vi "CO2FIX_GB19_Add455.vi"() -> ()   [LabVIEW 2018]
uses:
  <vilib>/DAQmx/read.llb/DAQmx Read (Analog DBL 1Chan 1Samp).vi
  <vilib>/DAQmx/create/channels.llb/DAQmx Create Channel (AI-Voltage-Basic).vi
  <vilib>/DAQmx/miscellaneous.llb/DAQmx Fill In Error Info.vi
  <vilib>/Utility/file.llb/Write Delimited Spreadsheet (DBL).vi
panel:
  out "Trans (Signal >275nm is more stable)":cluster{"Lumda":sgl[], "Intensity":sgl[]}(graph)
  out "< Thres":bool=TRUE
  out "number":u32=170738
  out "String":string="170738\r\n"
  out "Raw Data Graph 3":cluster{"Lumda":sgl[], "Intensity":sgl[]}(graph)
  in  "Save File":bool=TRUE
  in  "Save Background":bool
  out "> Thres":bool
  in  "stop":bool
  in  "Integration Time(ms)":i32=110
  in  "Average Times":i32=4
  in  "Wait Time":u32=120
  in  "UV300 Set":sgl=292000.0
  in  "UV340 Set":sgl=110378.0
  in  "Save ALL":bool=TRUE
  in  "file path (dialog if empty)":path=path "C:/Users/user/Desktop/CO2_Program/Data/0309/W_andMcd_New"
  in  "file path (dialog if empty) 2":path=path "C:/Users/user/Desktop/CO2_Program/Data/0309/W_and_Mcd_All_New"
  in  "Rate (ml/min)":dbl=0.003
  out "Dose Number":i32=1198
  in  "Pump Time":u32=1000
  out "Index":dbl=360.0
  in  "Wavelength":dbl=455.0
  in  "Pump RUN":bool
  in  "Connect the Pump":bool
  in  "Setting Tab":enum32{"UV and PL", "Range"}(tab)
  out "UV300":sgl(graph)=185217.0
  out "UV340":sgl(graph)=27758.75
  out "?":sgl=185217.0
  out "?":sgl=27758.75
  out "PL":dbl(graph)=0.15369048184948042
  out "?":dbl=0.15369048184948042 format="%0.2f"
  out "UV455 2":sgl=385808.3
  out "UV455":sgl(graph)=385808.3
  in  "Initial Wavelength 2":dbl=275.0
  out "Index 2":dbl=125.0
  in  "Final Wavelength":dbl=505.0
  out "Index 3":dbl=426.0
  out "subarray 2":sgl[](array[numeric])=[332.8669, 333.6288, 334.39072, 335.15262, 335.9145, 336.67633, 337.43814, 338.19995, 338.96173, 339.72348, 340.4852, 341.24692, 342.0086, 342.77026, 343.53192, 344.29355, 345.05515, 345.8167, 346.57825, 347.33978, 348.10126, 348.86273, 349.6242, 350.38562, 351.147, 351.9084]
  out "subarray":sgl[](array[numeric])=[290.1744, 290.93707, 291.6997, 292.46237, 293.225, 293.98764, 294.75027, 295.5129, 296.2755, 297.03812, 297.80072, 298.56332, 299.3259, 300.08847, 300.851, 301.6136, 302.37613, 303.13864, 303.90118, 304.6637, 305.42618, 306.1887, 306.95117, 307.71362, 308.47607, 309.23853]
  in  "index":i32=145
  in  "length 3":i32=26
  in  "index 2":i32=201
  in  "physical channels":tag="myDAQ1/ai0"
  out "Background":sgl[](graph)=[11662.829, 12200.412, 12741.526, 13266.624, 13764.132, 14239.703, 14700.305, 15169.1, 15633.125, 16080.848, 16526.568, 16951.803, 17352.846, 17742.307, 18115.617, 18481.635, 18861.121, 19228.037, 19607.826, 20033.656, 20506.39, 20975.314, 21429.824, 21874.693, 22314.486, 22720.926, 23099.477, 23464.29, 23812.91, 24120.67, 24402.24, 24671.984, 24942.217, 25128.393, 25328.764, 25352.076, 25260.271, 25075.955, 24881.014, 24785.152, 24827.955, 24950.078, 25146.15, 25347.043, 25523.666, 25693.074, 25799.213, 25776.885, 25635.168, 25390.854, 25115.197, 24923.48, 24850.783, 24866.639, 24948.094, 24974.553, 24984.9, 24962.344, 24914.252, 24755.438, 24523.752, 24313.99, 24132.727, 23955.791, 23793.834, 23694.123, 23663.645, 23690.838, 23774.723, 23913.729, 24066.088, 24197.506, 24283.953, 24334.453, 24349.229, 24376.02, 24419.385, 24459.86, 24472.574, 24419.55, 24302.516, 24156.85, 24001.873, 23888.658, 23819.984, 23787.754, 23826.557, 23969.12, 24233.43, 24581.705, 24935.51, 25101.64, 25095.82, 25118.697, 25217.166, 25398.553, 25656.426, 25987.393, 26384.482, 26612.795, 26693.918, 26686.576, 26673.998, 26773.516, 27020.361, 27379.266, 27767.031, 28061.688, 28225.52, 28304.275, 28338.377, 28412.365, 28553.605, 28743.72, 28936.129, 29089.033, 29184.336, 29222.68, 29278.357, 29416.11, 29634.06, 29921.674, 30173.553, 30232.85, 30100.656, 29836.76, 29570.885, 29519.438, 29756.2, 30166.668, 30678.26, 31253.81, 31798.094, 32115.113, 32270.998, 32535.479, 32940.16, 33297.176, 33591.727, 33730.51, 33711.863, 33752.2, 33593.383, 33535.496, 33506.03, 33496.426, 33561.37, 33725.746, 34031.348, 34486.812, 34979.957, 35071.03, 34906.305, 35122.027, 35674.387, 36218.492, 36514.16, 36119.66, 35296.406, 34884.29, 35104.91, 35851.824, 36744.855, 37013.312, 36519.266, 35533.914, 34533.707, 33783.926, 33529.125, 33507.043, 33761.26, 34125.36, 34354.758, 33803.387, 32718.762, 32014.986, 31773.3, 32030.799, 31726.107, 31596.922, 31384.887, 31393.861, 31548.842, 31469.758, 31146.816, 30741.807, 30337.123, 30063.309, 29974.361, 29922.512, 30067.191, 30719.6, 31695.77, 32920.945, 33695.24, 33394.07, 32401.562, 31569.3, 30980.309, 30304.057, 29715.104, 29526.53, 29929.428, 31339.666, 33072.6, 33885.43, 33322.734, 31445.363, 30226.885, 30152.033, 30646.63, 30937.982, 30534.053, 30046.96, 29539.832, 29029.887, 28704.307, 28765.17, 29236.066, 30154.299, 31222.639, 31898.865, 32050.398, 31853.746, 31434.635, 30982.043, 30593.57, 30154.084, 29726.898, 29487.102, 29371.229, 29195.447, 28703.057, 28216.209, 27783.318, 27229.06, 26700.953, 26456.951, 26509.146, 26732.828, 26917.287, 27316.756, 27877.488, 28221.094, 28203.2, 27723.234, 26970.273, 25911.797, 25373.816, 25795.814, 26985.47, 27935.127, 28164.598, 27135.84, 25322.652, 23791.945, 22817.662, 21753.3, 20725.24, 20196.85, 20215.668, 20613.348, 21187.29, 21629.316, 21783.09, 21561.031, 21078.72, 20720.355, 20649.633, 20746.46, 20994.38, 21363.48, 21437.719, 21286.775, 21083.664, 20873.533, 22341.213, 30386.02, 42265.0, 47372.523, 43005.14, 30858.705, 22305.854, 19230.033, 18336.748, 18041.25, 17642.873, 17564.633, 17787.107, 17785.61, 17619.354, 17703.818, 17906.27, 17665.78, 17110.701, 16657.889, 16782.773, 16929.34, 17048.264, 17154.547, 17162.465, 17056.4]
  in  "index 3":i32=355
  in  "length":i32=15
  out "subarray 3":sgl[](array[numeric])=[449.83356, 450.5899, 451.34622, 452.1025, 452.8587, 453.6149, 454.371, 455.12708, 455.8831, 456.63907, 457.395, 458.15088, 458.9067, 459.66248, 460.4182]
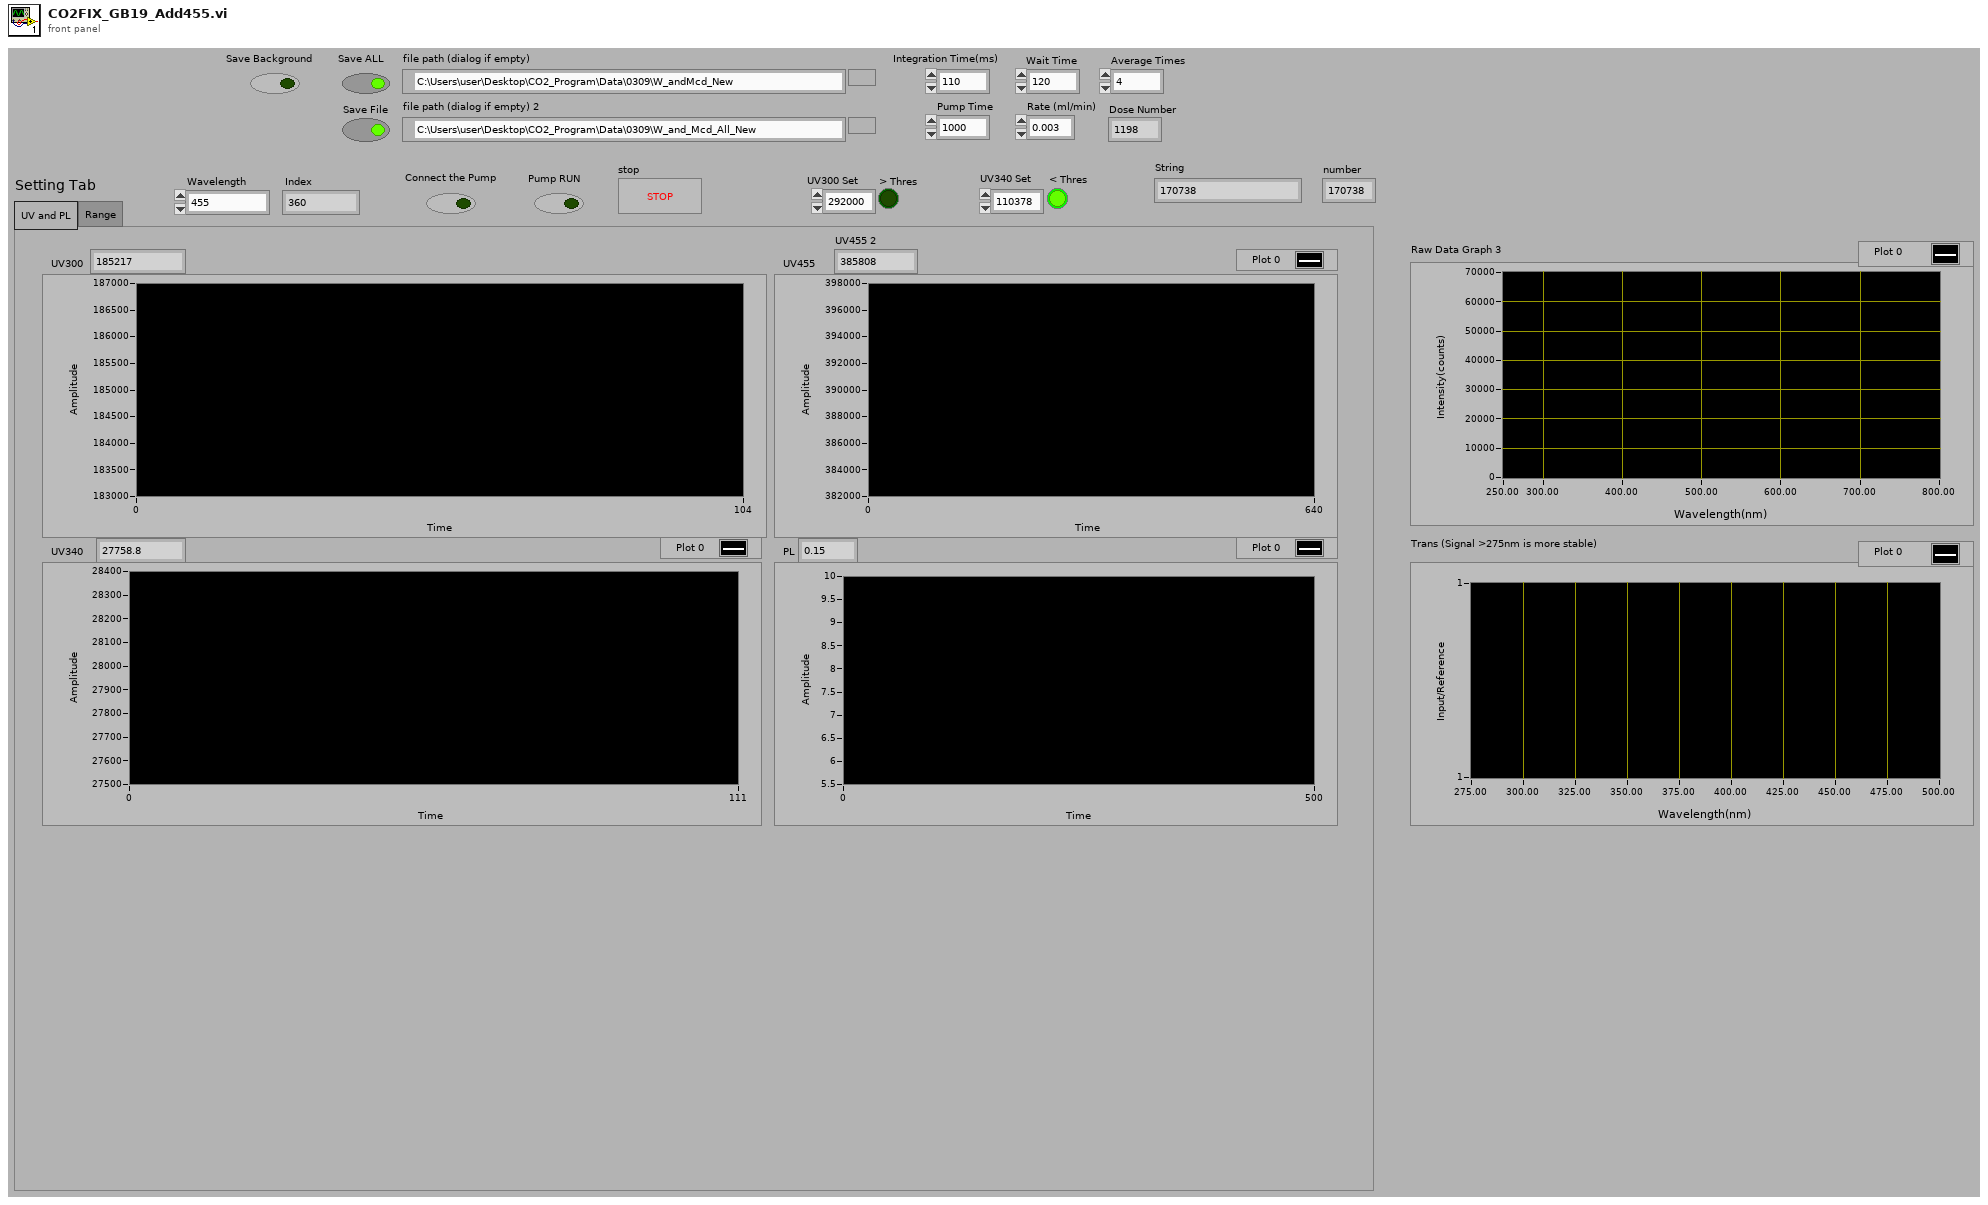
[diagram p1: front panel]
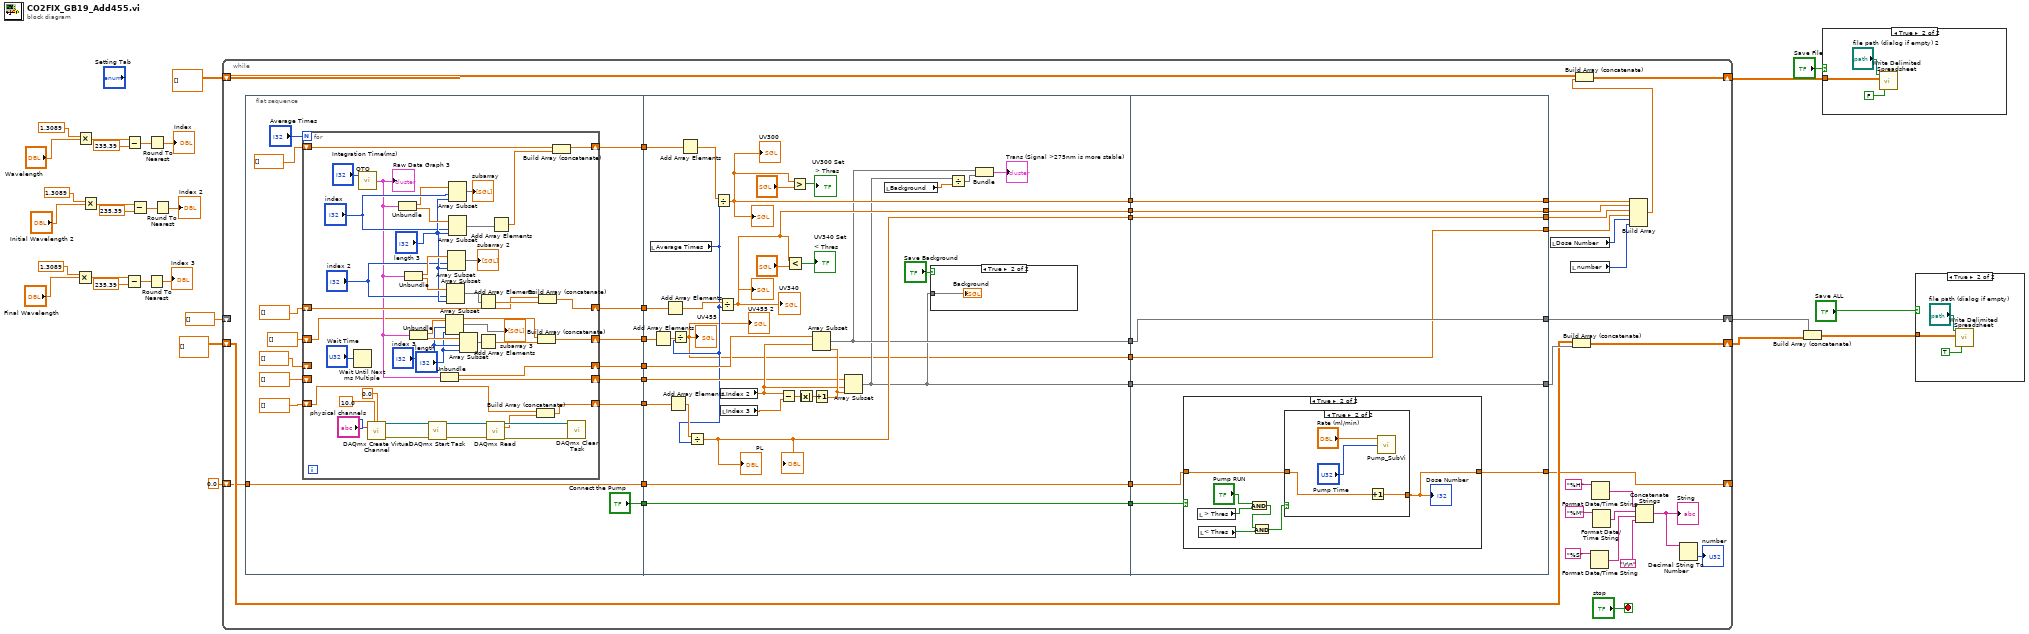
[diagram p0: block diagram]
diagram:
  n1 = Multiply(x=1.3089, y="Final Wavelength") -> (x*y=w12:dbl)
  n2 = Multiply(x=1.3089, y="Wavelength") -> (x*y=w27:dbl)
  n3 = Multiply(x=1.3089, y="Initial Wavelength 2") -> (x*y=w18:dbl)
  n4 = Subtract(x=w12, y=235.39) -> (x-y=w11:dbl)
  n5 = Subtract(x=w27, y=235.39) -> (x-y=w26:dbl)
  n6 = Subtract(x=w18, y=235.39) -> (x-y=w17:dbl)
  n7 = Round To Nearest(number=w11) -> (nearest integer value=→"Index 3":dbl)
  n8 = Round To Nearest(number=w26) -> (nearest integer value=→"Index":dbl)
  n9 = Round To Nearest(number=w17) -> (nearest integer value=→"Index 2":dbl)
  n10 = while {
    shift-right: [w49] -> w3
    shift-left: sgl[][] [] -> [w47]
    shift-right: [w55] -> w20
    shift-left: sgl[][] [] -> [w69]
    shift-right: [w48] -> w4
    shift-left: sgl[] [] -> [_]
    shift-right: [w46] -> _
    shift-left: 0.0 -> [w45]
    stop <- "stop" stop-if-true
    n11 = flat-sequence {
      tunnel: [w78] -> w67
      tunnel: [w77] -> w66
      tunnel: [w76] -> w65
      tunnel: ["Connect the Pump"] -> w61
      tunnel: [w74] -> w54
      tunnel: [w73] -> w53
      tunnel: w45 -> [w72]
      tunnel: [w72] -> w44
      tunnel: [w70] -> w33
      tunnel: w67 -> [w146]
      tunnel: w66 -> [w145]
      tunnel: w65 -> [w144]
      tunnel: [w148] -> w64
      tunnel: [w147] -> w63
      tunnel: [w143] -> w62
      tunnel: w61 -> [w143]
      tunnel: [w142] -> w58
      tunnel: w54 -> [w141]
      tunnel: w53 -> [w140]
      tunnel: [w134] -> w51
      tunnel: [w136] -> w50
      tunnel: w44 -> [w139]
      tunnel: [w139] -> w43
      tunnel: w33 -> [w131]
      tunnel: [w128] -> w30
      tunnel: [w168] -> w60
      tunnel: [w169] -> w59
      tunnel: w64 -> [w169]
      tunnel: w63 -> [w168]
      tunnel: w62 -> [w167]
      tunnel: [w166] -> w57
      tunnel: w58 -> [w166]
      tunnel: [w165] -> w52
      tunnel: w51 -> [w165]
      tunnel: w50 -> [w164]
      tunnel: [w164] -> w48
      tunnel: [w163] -> w46
      tunnel: w43 -> [w162]
      tunnel: w30 -> [w161]
      tunnel: [w161] -> w29
      frame #0 {
        n12 = for {
          N: "Average Times" -> [_]
          shift-right: [w121] -> w78
          shift-left: sgl[] [] -> [w120]
          shift-right: [w117] -> w76
          shift-left: sgl[] [] -> [w116]
          shift-right: [w113] -> w73
          shift-left: sgl[] [] ("Intensity") -> [_]
          shift-right: [w112] -> w74
          shift-left: sgl[] [] -> [_]
          shift-right: [w96] -> w77
          shift-left: dbl[] [] -> [w95]
          shift-right: [w90] -> w70
          shift-left: sgl[] [] -> [w89]
          n13 = Wait Until Next ms Multiple(millisecond multiple="Wait Time") -> ()  [unwired: 1 out]
          n14 = call "OTO.vi"("Integration Time(ms)"="Integration Time(ms)") -> ("Raw Data Graph"=w93:cluster{"Lumda":sgl[], "Intensity":sgl[]})  [unwired: 2 in]
          "Raw Data Graph 3" <- w93
          n15 = call-poly <vilib>:"DAQmx Create Virtual Channel.vi"("maximum value"=10.0, "minimum value"=0.0, "physical channels"="physical channels") -> ("task out"=w104:refnum<k21>, "error out"=w101:errorcluster)  [unwired: 11 in]
          n16 = Unbundle(w93) -> ("Lumda"=w109:sgl[], "Intensity"=w126:sgl[])
          n17 = Unbundle(w93) -> ("Lumda"=w125:sgl[], "Intensity"=w124:sgl[])
          n18 = Unbundle(w93) -> ("Lumda"=w87:sgl[], "Intensity"=w92:sgl[])
          n19 = call <vilib>:"DAQmx Start Task.vi"("task/channels in"=w104, "error in"=w101) -> ("task out"=w105:refnum<k21>, "error out"=w102:errorcluster)  [unwired: 12 in]
          n20 = Unbundle(w93) -> ("Lumda"=w112:sgl[], "Intensity"=w113:sgl[])
          n21 = Array Subset(array=w87, index="index 3", length="length") -> (→"subarray 3":sgl[])
          n22 = Array Subset(array=w124, index="index 2", length="length 3") -> (w114:sgl[])
          n23 = Array Subset(array=w125, index="index 2", length="length 3") -> (→"subarray 2":sgl[])
          n24 = Array Subset(array=w126, index="index", length="length 3") -> (w119:sgl[])
          n25 = Array Subset(array=w109, index="index", length="length 3") -> (→"subarray":sgl[])
          n26 = Array Subset(array=w92, index="index 3", length="length") -> (w94:sgl[])
          n27 = Add Array Elements(numeric array=w114) -> (sum=w118:sgl)
          n28 = Add Array Elements(numeric array=w94) -> (sum=w91:sgl)
          n29 = call-poly <vilib>:"DAQmx Read.vi"("task/channels in"=w105, "error in"=w102) -> ("task out"=w106:refnum<k21>, "data"=w97:dbl, "error out"=w103:errorcluster)  [unwired: 11 in]
          n30 = Add Array Elements(numeric array=w119) -> (sum=w115:sgl)
          n31 = Build Array (concatenate)(w95, w97) -> (w96:dbl[])
          n32 = Build Array (concatenate)(w89, w91) -> (w90:sgl[])
          n33 = Build Array (concatenate)(w116, w118) -> (w117:sgl[])
          n34 = Build Array (concatenate)(w120, w115) -> (w121:sgl[])
          n35 = call <vilib>:"DAQmx Clear Task.vi"("task in"=w106, "error in"=w103) -> ()  [unwired: 13 in, 1 out]
        }
      }
      frame #1 {
        n36 = local read "Average Times"() -> (w129:i32)
        n37 = Add Array Elements(numeric array=w131) -> (sum=w130:sgl)
        n38 = Add Array Elements(numeric array=w144) -> (sum=w149:sgl)
        n39 = Add Array Elements(numeric array=w145) -> (sum=w159:dbl)
        n40 = Divide(x=w130, y=w129) -> (x/y=w128:sgl)
        "UV455" <- w128
        "UV455 2" <- w128
        n41 = Add Array Elements(numeric array=w146) -> (sum=w150:sgl)
        n42 = Divide(x=w159, y=w129) -> (x/y=w142:dbl)
        "?" <- w142
        "PL" <- w142
        n43 = Divide(x=w150, y=w129) -> (x/y=w147:sgl)
        "UV300" <- w147
        "?" <- w147
        n44 = Divide(x=w149, y=w129) -> (x/y=w148:sgl)
        "UV340" <- w148
        "?" <- w148
        n45 = local read "Index 2"() -> (w157:dbl)
        n46 = local read "Index 3"() -> (w153:dbl)
        n47 = Subtract(x=w157, y=w153) -> (x-y=w152:dbl)
        n48 = Less?(x=w148, y="UV340 Set") -> (x < y?=→"< Thres":bool)
        n49 = Greater?(x=w147, y="UV300 Set") -> (0:→"> Thres":bool)
        n50 = Absolute Value(x=w152) -> (abs(x)=w151:dbl)
        n51 = Increment(x=w151) -> (x+1=w158:dbl)
        n52 = Array Subset(array=w141, index=w157, length=w158) -> (w136:sgl[])
        n53 = Array Subset(array=w140, index=w157, length=w158) -> (w134:sgl[])
        n54 = local read "Background"() -> (w135:sgl[])
        n55 = case shown="True" "Save Background" {
          tunnel: w134 -> [_ w160]
          frame False {
          }
          frame True {
            "Background" <- w160
          }
        }
        n56 = Divide(x=w134, y=w135) -> (x/y=w133:sgl[])
        n57 = Bundle(w136, w133) -> (→"Trans (Signal >275nm is more stable)":cluster{sgl[], sgl[]})  [unwired: 1 in]
      }
      frame #2 {
        n58 = case shown="True" w167 {
          tunnel: [w170 w177] -> w163
          tunnel: w162 -> [w170 w176]
          frame False {
          }
          frame True {
            n59 = local read "> Thres"() -> (w174:bool)
            n60 = local read "< Thres"() -> (w171:bool)
            n61 = And(x="Pump RUN", y=w174) -> (x .and. y?=w173:bool)
            n62 = And(x=w173, y=w171) -> (x .and. y?=w172:bool)
            n63 = case shown="True" w172 {
              tunnel: [w178 w182] -> w177
              tunnel: w176 -> [w178 w179]
              frame False {
              }
              frame True {
                n64 = Increment(x=w179) -> (x+1=w182:dbl)
                n65 = call "Pump_SubVi.vi"("Each Pumping Time"="Pump Time", "rate (ml/min)"="Rate (ml/min)") -> ()  [unwired: 1 in]
              }
            }
            "Dose Number" <- w177
          }
        }
      }
    }
    n66 = local read "Dose Number"() -> (w32:i32)
    n67 = local read "number"() -> (w31:u32)
    n68 = Build Array (concatenate)(w47, w52) -> (w49:sgl[][])
    n69 = Format Date/Time String(time format string (%c)="%S") -> (date/time string=w37:string)  [unwired: 2 in]
    n70 = Format Date/Time String(time format string (%c)="%H") -> (date/time string=w39:string)  [unwired: 2 in]
    n71 = Format Date/Time String(time format string (%c)="%M") -> (date/time string=w38:string)  [unwired: 2 in]
    n72 = Build Array(w60, w59, w57, w29, w32, w31) -> (w56:dbl[])
    n73 = Build Array (concatenate)(w69, w56) -> (w55:dbl[][])
    n74 = Concatenate Strings(w39, w38, w37, "\r\n") -> (w35:string)
    "String" <- w35
    n75 = Decimal String To Number(string=w35) -> (number=→"number":i32)  [unwired: 2 in, 1 out]
  }
  n76 = Build Array (concatenate)(w4, w3) -> (w5:sgl[][])
  n77 = case shown="True" "Save File" {
    tunnel: w20 -> [_ w183]
    frame False {
    }
    frame True {
      n78 = call-poly <vilib>:"Write Delimited Spreadsheet.vi"("file path (dialog if empty)"="file path (dialog if empty) 2", "2D data"=w183, "transpose? (no:F)"=FALSE) -> ()  [unwired: 11 in, 2 out]
    }
  }
  n79 = case shown="True" "Save ALL" {
    tunnel: w5 -> [_ w186]
    frame False {
    }
    frame True {
      n80 = call-poly <vilib>:"Write Delimited Spreadsheet.vi"("file path (dialog if empty)"="file path (dialog if empty)", "2D data"=w186, "transpose? (no:F)"=TRUE) -> ()  [unwired: 11 in, 2 out]
    }
  }
